vi "user input.vi"(8 "error in":errorcluster) -> (0 "error out":errorcluster, 3 "Inputs from system":T1)   [LabVIEW 2014]
uses:
  input user data.ctl
  DAQmx Watchdog runtime.lvclass
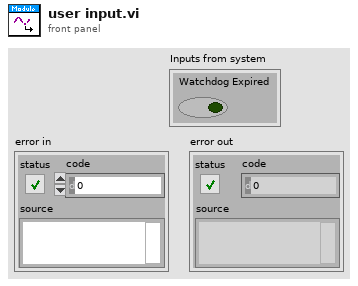
[diagram p1: front panel]
types:
  T1 = typedef "DAQmx Watchdog runtime.lvclass/input user data.ctl" = cluster{"Watchdog Expired":bool}
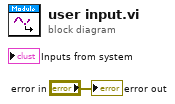
[diagram p0: block diagram]
diagram:
  "error out" <- "error in"
